vi "Globals.vi"() -> ()   [LabVIEW 2013]
panel:
  out "Slide":dbl
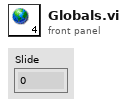
[diagram p1: front panel]
diagram:
